vi "05 - Exemple - Wrapping In lvclass.vi"() -> ()   [LabVIEW 2016]
uses:
  Library/Skeleton/Skeleton.lvclass
panel:
  out "Sum":i64
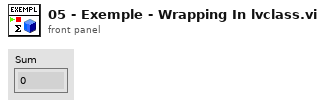
[diagram p1: front panel]
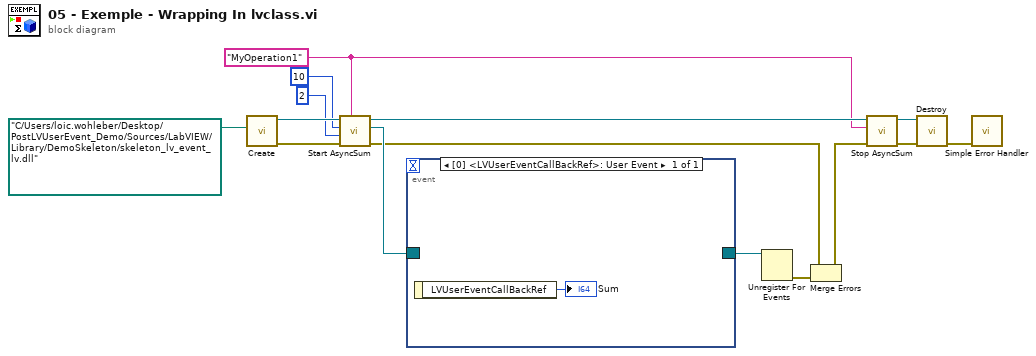
[diagram p0: block diagram]
diagram:
  w2 = "MyOperation1" ("Opeation")
  n1 = call "Create.vi"("DLL path"=path "C:/Users/loic.wohleber/Desktop/PostLVUserEvent_Demo/Sources/LabVIEW/Library/DemoSkeleton/skeleton_lv_event_lv.dll") -> ("error out"=w14:errorcluster, "Skeleton out"=w15:refnum<class "Skeleton.lvclass">)  [unwired: 9 in]
  n2 = call "Start AsyncSum.vi"("Opeation"=w2, "error in (no error)"=w14, "B"=2 ("A"), "A"=10, "Skeleton in"=w15) -> ("error out"=w5:errorcluster, "AsyncSum Event Register"=w8:refnum<event-registration>, "Skeleton out"=w10:refnum<class "Skeleton.lvclass">)  [unwired: 4 in]
  n3 = event shown="[0] <LVUserEventCallBackRef>: User Event" {
    selector: w8 -> [_]
    dyn-events: [_] -> w7
    timeout: _ -> [_]
    event User Event {
      n4 = event-data() -> ("LVUserEventCallBackRef"=→"Sum":i64)  [unwired: 1 in]
    }
  }
  n5 = Unregister For Events(event registration refnum=w7) -> (error out=w6:errorcluster)  [unwired: 1 in]
  n6 = Merge Errors(w5, w6) -> (w4:errorcluster)
  n7 = call "Stop AsyncSum.vi"("error in (no error)"=w4, "Opeation"=w2, "Skeleton in"=w10) -> ("error out"=w11:errorcluster, "Skeleton out"=w9:refnum<class "Skeleton.lvclass">)  [unwired: 7 in]
  n8 = call "Destroy.vi"("error in (no error)"=w11, "Skeleton in"=w9) -> ("error out"=w3:errorcluster)  [unwired: 9 in]
  n9 = call <vilib>:"Simple Error Handler.vi"("error in (no error)"=w3) -> ()  [unwired: 4 in, 5 out]
